vi "Read Data Type.vi"(8 "error in (no error)":errorcluster, 11 "OnChange_Boolean in":refnum<class "OnChangeNotifier_String.lvclass">) -> (0 "error out":errorcluster, 2 "Abs_String.lvclass":refnum<class "Abs_String.lvclass">, 3 "OnChange_Boolean out":refnum<class "OnChangeNotifier_String.lvclass">)   [LabVIEW 2021, in "OnChangeNotifier_String.lvclass"]
uses:
  OnChangeNotifier_String.lvclass
  <vilib>/TSA/Abstract Data Classes/Abs_Types/String/Abs_String.lvclass
  OnChangeNotifier_String.lvclass/OnChangeNotifier_String.ctl
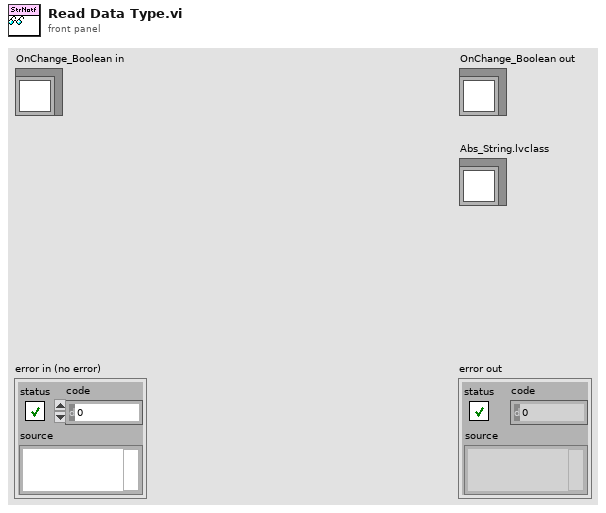
[diagram p1: front panel]
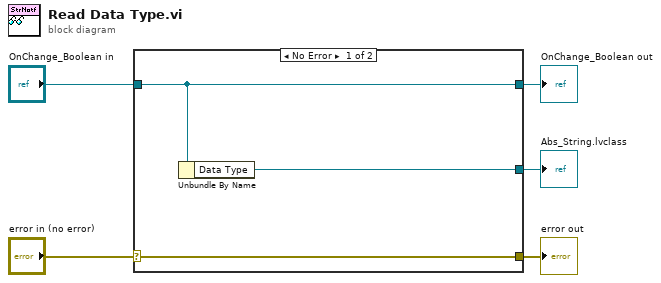
[diagram p0: block diagram]
diagram:
  n1 = case shown="No Error" "error in (no error)" {
    selector: "error in (no error)" -> [w8 w9]
    tunnel: [w8 w9] -> w4
    tunnel: [w7 w10] -> w2
    tunnel: "OnChange_Boolean in" -> [w7 w10]
    tunnel: [w6 _] -> w1
    frame No Error {
      n2 = Unbundle By Name(w7) -> ("Data Type"=w6:refnum<class "Abs_String.lvclass">)
    }
    frame Error {
    }
  }
  "error out" <- w4
  "OnChange_Boolean out" <- w2
  "Abs_String.lvclass" <- w1
